vi "Configure Limit Setting.vi"(7 "Limit Value Type (0: Volts)":i32(ring) items=["Volts", "Current"], 8 "error in (no error)":errorcluster, 9 "- Limit Value (-5)":dbl=-5.0, 10 "+ Limit Value (5)":dbl=5.0, 11 "VISA resource name":refnum<visa-resource-name>) -> (0 "error out":errorcluster, 3 "VISA resource name out":refnum<visa-resource-name>)   [LabVIEW 2012, in "Fluke 5080.lvlib"]
doc: "Configures the limitation of output."
uses:
  <instrlib>/Fluke 5080/Fluke 5080.lvlib
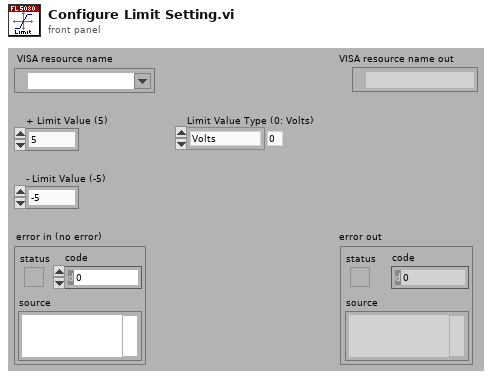
[diagram p1: front panel]
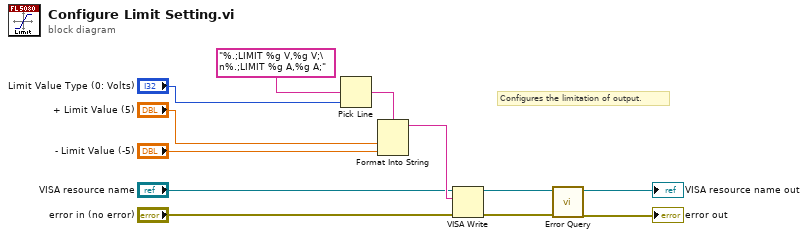
[diagram p0: block diagram]
diagram:
  # "Configures the limitation of output."
  n1 = Pick Line(multi-line string="%.;LIMIT %g V,%g V;\n%.;LIMIT %g A,%g A;", line index="Limit Value Type (0: Volts)") -> (output string=w1:string)  [unwired: 1 out]
  n2 = Format Into String(format string=w1, "+ Limit Value (5)", "- Limit Value (-5)") -> (resulting string=w10:string)  [unwired: 2 in, 1 out]
  n3 = VISA Write(VISA resource name="VISA resource name", write buffer=w10, error in (no error)="error in (no error)") -> (VISA resource name out=w7:refnum<visa-resource-name>, error out=w6:errorcluster)  [unwired: 1 out]
  n4 = call <instrlib>:"Error Query.vi"("error in (no error)"=w6, "VISA resource name"=w7) -> ("error out"=→"error out":errorcluster, "VISA resource name out"=→"VISA resource name out":refnum<visa-resource-name>)  [unwired: 8 out]
